vi "Send WG commands and wait for answers.vi"(0 "System no.":i32=1 min=1 max=4 step=1, 3 "Command array":string[](array[string]), 5 "error in":errorcluster) -> (14 "Controller error":bool, 19 "error out":errorcluster)   [LabVIEW 2020]
doc: "This VI sends the wave generator commands from Command array to the given system and waits for the controller to reply. Use WGWaveEditor_with_parameter.vi, or use the WGWaveEditorl_call_Editor.vi, and WGWaveEditor_read_commands.vi to receive the strings for Command array from WGWaveEditor.dll. Controller error is TRUE if selected system reports an error code which is not zero."
panel:
  # "This vi sends the wave generator commands from \"Command array\" to the given\nsystem and waits for the controller to reply. Use WGWaveEditor_with_parameter.vi, or \nuse the WGWaveEditor_call_Editor.vi and  WGWaveEditor_read_commands.vi. to receive\nthe strings for \"Command array\" from  WGWaveEditor.dll."
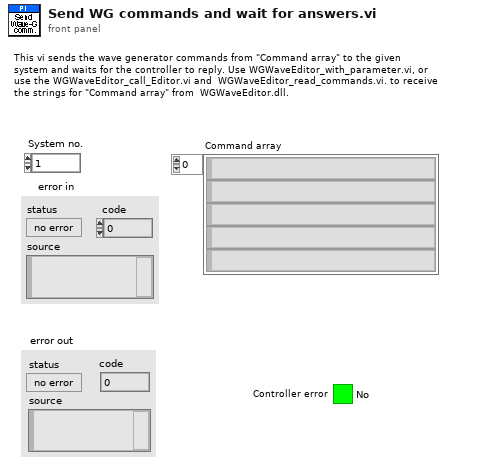
[diagram p1: front panel]
types:
  T1 = enum16{"Disable error check", "Force error check", "Use global settings"}
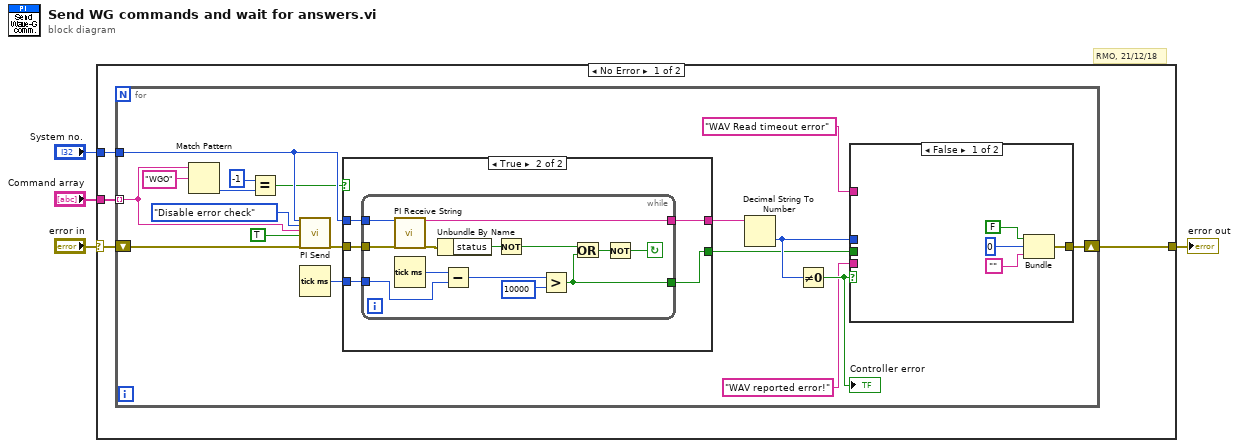
[diagram p0: block diagram]
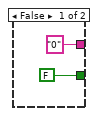
[diagram p2: hidden frame]
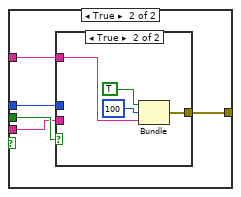
[diagram p3: hidden frame]
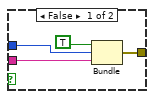
[diagram p4: hidden frame]
diagram:
  # "RMO, 21/12/18"
  n1 = case shown="No Error" "error in" {
    selector: "error in" -> [w5 w64]
    tunnel: [w8 w64] -> w4
    tunnel: "System no." -> [w7 _]
    tunnel: "Command array" -> [w6 _]
    frame No Error {
      n2 = for {
        shift-right: [w18] -> w8
        shift-left: w5 -> [w19]
        tunnel: w7 -> [w16]
        tunnel: w6 -> [w14] mode=indexing
        n3 = Match Pattern(string=w14, regular expression="WGO") -> (offset past match=w12:i32)  [unwired: 4 out]
        n4 = Equal?(x=-1, y=w12) -> (x = y?=w10:bool)
        n5 = call "PI Send.vi"("System no."=w16, "Error check settings"=T1."Disable error check", "String to send"=w14, "Attach termination char.?"=TRUE ("Attach Linefeed?"), "error in"=w19) -> ("error out"=w24:errorcluster)  [unwired: 1 in, 13 out]
        n6 = Tick Count (ms)() -> (millisecond timer value=w25:u32)
        n7 = case shown="True" w10 {
          tunnel: w25 -> [_ w33]
          tunnel: w24 -> [_ w32]
          tunnel: ["0" ("String read") w31] -> w17
          tunnel: w16 -> [_ w30]
          tunnel: [FALSE w29] -> w15
          frame False {
          }
          frame True {
            n8 = while {
              tunnel: [w34] -> w29
              tunnel: [w35] -> w31
              tunnel: w30 -> [w36]
              tunnel: w32 -> [w37]
              tunnel: w33 -> [w38]
              stop <- w39 continue-if-true
              n9 = call "PI Receive String.vi"("System no."=w36, "error in"=w37) -> ("String read"=w35:string, "error out"=w46:errorcluster)  [unwired: 1 in, 15 out]
              n10 = Tick Count (ms)() -> (millisecond timer value=w44:u32)
              n11 = Unbundle By Name(w46) -> ("status"=w45:bool)
              n12 = Subtract(x=w44, y=w38) -> (x-y=w43:u32)
              n13 = Not(x=w45) -> (.not. x?=w41:bool)
              n14 = Greater?(x=w43, y=u32 10000) -> (0:w34:bool)
              n15 = Or(x=w41, y=w34) -> (x .or. y?=w40:bool)
              n16 = Not(x=w40) -> (.not. x?=w39:bool)
            }
          }
        }
        n17 = Decimal String To Number(string=w17) -> (number=w21:i32)  [unwired: 3 out]
        n18 = Not Equal To 0?(x=w21) -> (x != 0?=w23:bool)
        "Controller error" <- w23
        n19 = case shown="False" w23 {
          tunnel: w15 -> [_ w55]
          tunnel: "WAV Read timeout error" -> [_ w54]
          tunnel: w21 -> [_ w53]
          tunnel: "WAV reported error!" -> [_ w52]
          tunnel: [w47 w51] -> w18
          frame False {
            n20 = Bundle(FALSE, 0, "") -> (w47:errorcluster)  [unwired: 1 out]
          }
          frame True {
            n21 = case shown="True" w55 {
              tunnel: w54 -> [_ w61]
              tunnel: w53 -> [w58 _]
              tunnel: w52 -> [w57 _]
              tunnel: [w56 w60] -> w51
              frame False {
                n22 = Bundle(TRUE, w58, w57) -> (w56:errorcluster)  [unwired: 1 out]
              }
              frame True {
                n23 = Bundle(TRUE, 100, w61) -> (w60:errorcluster)  [unwired: 1 out]
              }
            }
          }
        }
      }
    }
    frame Error {
    }
  }
  "error out" <- w4
